vi "Read Push Time.vi"(8 "error in (no error)":errorcluster, 11 "cRIO-CO2 in":refnum<class "cRIO-CO2.lvclass">) -> (0 "error out":errorcluster, 1 "Push Time (sec)":dbl, 3 "cRIO-CO2 out":refnum<class "cRIO-CO2.lvclass">)   [LabVIEW 2015, in "cRIO-Carbondioxide.lvlib" / "cRIO-CO2.lvlib" / "cRIO-CO2.lvclass"]
uses:
  cRIO-CO2.lvclass
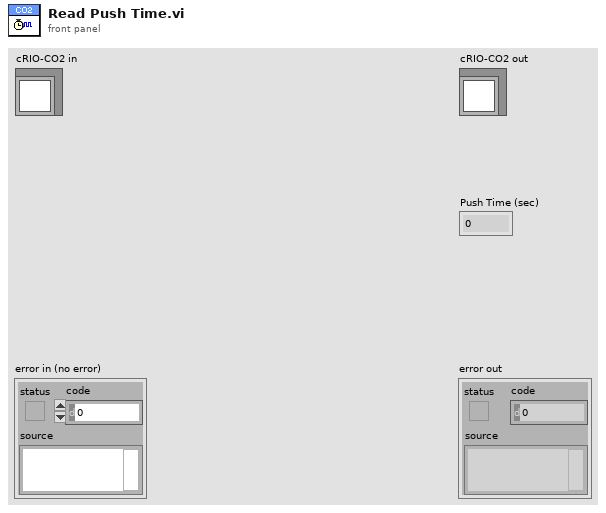
[diagram p1: front panel]
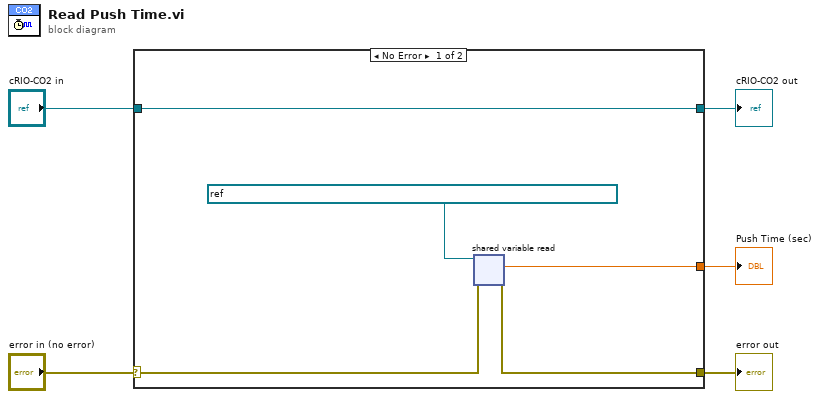
[diagram p0: block diagram]
diagram:
  n1 = case shown="No Error" "error in (no error)" {
    selector: "error in (no error)" -> [w9 w12]
    tunnel: [w8 w12] -> w4
    tunnel: [w10 w11] -> w2
    tunnel: "cRIO-CO2 in" -> [w10 w11]
    tunnel: [w7 _] -> w1
    frame No Error {
      n2 = shared-variable-read(refnum<k21> "ni.var.psp://cRIO-Carbondioxide/AMS Gas SHV/Sample Push/Push Time" ("shared variable refnum in"), w9) -> (w8:errorcluster, w7:dbl)  [unwired: 1 out]
    }
    frame Error {
    }
  }
  "error out" <- w4
  "cRIO-CO2 out" <- w2
  "Push Time (sec)" <- w1
